vi "maze_v4.vi"   [LabVIEW 2012]
uses:
  <vilib>/NXT/Subs/MotorOutput.ctl
  <vilib>/NXT/Dual Mode Library/Sound/Tone.vi
types:
  T1 = typedef "MotorOutput.ctl" = u8
  T2 = typedef "LVHSConnector.ctl" = cluster{"Hardware":string, "Flattened String":string}
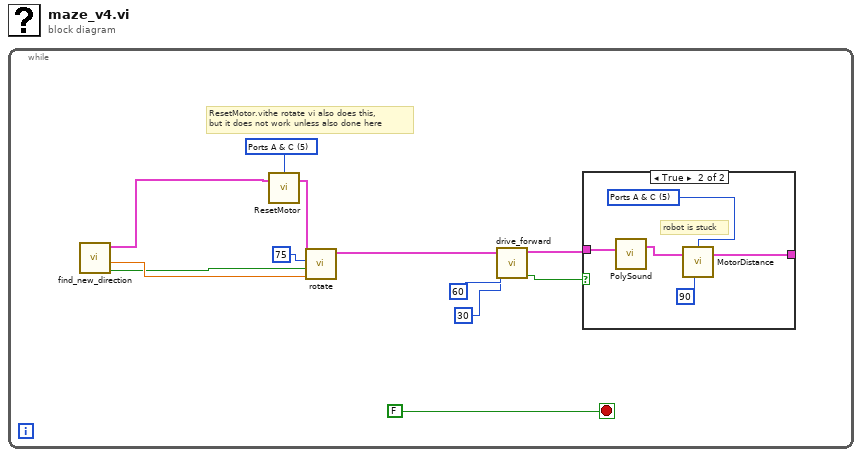
[diagram p0: block diagram]
diagram:
  n1 = while {
    stop <- FALSE stop-if-true
    w12 = T1 5 items=["Port A"=0, "Port B"=1, "Port C"=2, "Ports A & B"=4, "Ports A & C"=5, "Ports B & C"=6, "All Ports"=3] ("Port (All Ports)")
    # "ResetMotor.vithe rotate vi also does this,\nbut it does not work unless also done here"
    n2 = call "find_new_direction.vi"() -> ("right(T)/left(F)"=w9:bool, "angle"=w10:dbl, "NXT 2"=w2:T2)  [unwired: 9 in]
    n3 = call <vilib>:"ResetMotor.vi"("NXT"=w2, "Port (All Ports)"=w12) -> ("NXT"=w11:T2)  [unwired: 2 in]
    n4 = call "rotate.vi"("degrees to  rotate"=w10, "right(T)/left(F)"=w9, "power"=u16 75, "NXT 2"=w11) -> ("NXT"=w8:T2)  [unwired: 7 in]
    n5 = call "drive_forward.vi"("min distance"=u16 30 ("power"), "power"=u16 60, "NXT"=w8) -> ("stuck"=w4:bool, "NXT 2"=w3:T2)  [unwired: 7 in]
    n6 = case shown="True" w4 {
      tunnel: w3 -> [w13 w18]
      tunnel: [w13 w15] -> _
      frame False {
      }
      frame True {
        w14 = T1 5 items=["Port A"=0, "Port B"=1, "Port C"=2, "Ports A & B"=4, "Ports A & C"=5, "Ports B & C"=6, "All Ports"=3] ("Output Port (All Ports)")
        # "robot is stuck"
        n7 = call-poly <vilib>:"PolySound.vi"("NXT"=w18) -> ("NXT"=w17:T2)  [unwired: 3 in]
        n8 = call <vilib>:"MotorDistance.vi"("Angle of Rotation (360)"=90, "NXT"=w17, "Output Port (All Ports)"=w14) -> ("NXT"=w15:T2)  [unwired: 1 in]
      }
    }
  }
